vi "Config to String.vi"(8 "error in (no error)":errorcluster, 11 "queue in":T1) -> (0 "error out":errorcluster, 2 "String":string, 3 "queue out":T1)   [LabVIEW 2020, in "NI_LVConfig.lvlib"]
uses:
  NI_LVConfig.lvlib
  Config Queue.ctl
  Config Data.ctl
  Section.ctl
  8.6CompatibleGlobalVar.vi
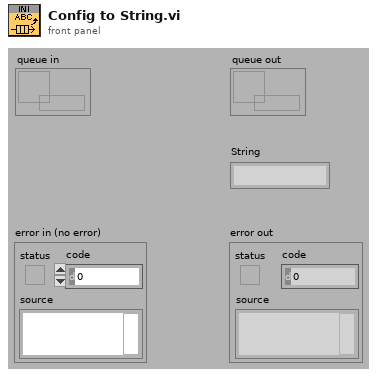
[diagram p1: front panel]
types:
  T1 = typedef "NI_LVConfig.lvlib/Config Queue.ctl" = refnum<queue>
  T2 = typedef "NI_LVConfig.lvlib/Config Data.ctl" = cluster{"sections":T3[], "path":path, "dirty":bool}
  T3 = typedef "NI_LVConfig.lvlib/Section.ctl" = cluster{"name":string, "comment":string, "kvc":string[][]}
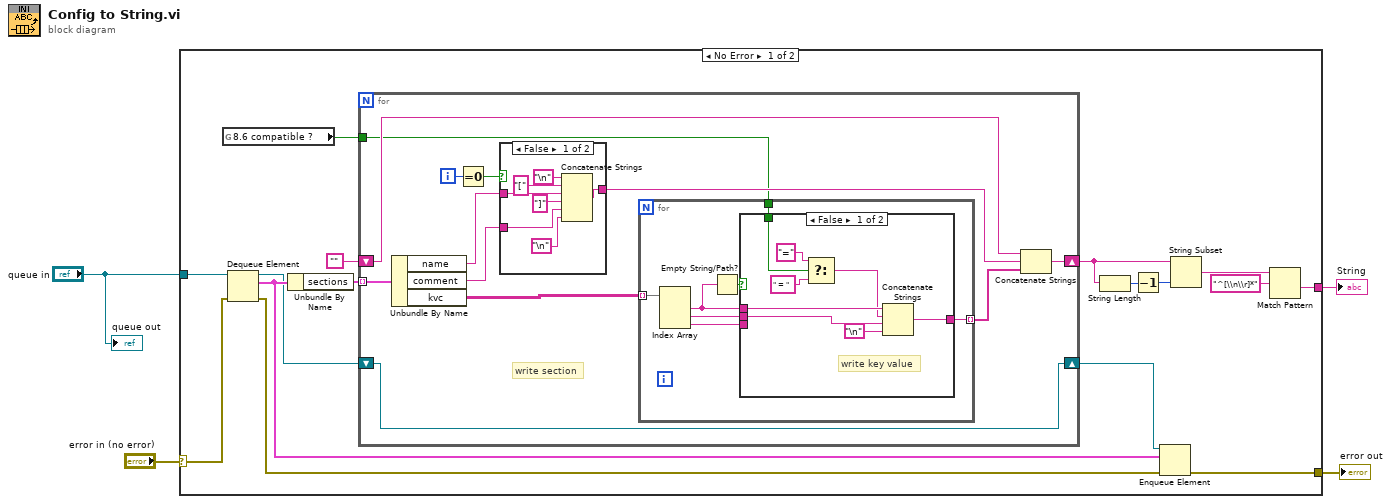
[diagram p0: block diagram]
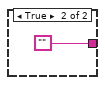
[diagram p2: hidden frame]
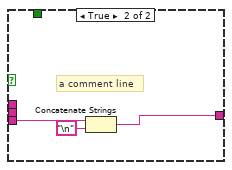
[diagram p3: hidden frame]
diagram:
  n1 = case shown="No Error" "error in (no error)" {
    selector: "error in (no error)" -> [w18 w59]
    tunnel: "queue in" -> [w19 _]
    tunnel: [w15 _] -> w4
    tunnel: [w9 w59] -> w2
    frame No Error {
      n2 = global read "8.6CompatibleGlobalVar.vi" "8.6 compatible ?"() -> (w5:bool)
      n3 = Dequeue Element(queue=w19, error in (no error)=w18) -> (queue out=w7:T1, element=w8:T2, error out=w10:errorcluster)  [unwired: 1 in, 1 out]
      n4 = Unbundle By Name(w8) -> ("sections"=w20:T3[])
      n5 = for {
        tunnel: w20 -> [w32] mode=indexing
        shift-right: [w30] -> w12
        shift-left: "" -> [w29]
        shift-right: [w22] -> w6
        shift-left: w7 -> [w22]
        tunnel: w5 -> [w21]
        i -> [w27]
        # "write section"
        n6 = Unbundle By Name(w32) -> ("name"=w28:string, "comment"=w23:string, "kvc"=w24:string[][])
        n7 = Equal To 0?(x=w27) -> (x = 0?=w26:bool)
        n8 = case shown="False" w26 {
          tunnel: w28 -> [w37 _]
          tunnel: [w36 ""] -> w31
          tunnel: w23 -> [w34 _]
          frame False {
            n9 = Concatenate Strings("\n", "[" ("string"), w37, "]" ("string"), w34, "\n") -> (w36:string)
          }
          frame True {
          }
        }
        n10 = for {
          tunnel: w24 -> [w47] mode=indexing
          tunnel: [w44] -> w25 mode=indexing
          tunnel: w21 -> [w41]
          n11 = Index Array(array=w47) -> (element #1=w42:string, element #2=w43:string, element #3=w45:string)  [unwired: 3 in]
          n12 = Empty String/Path?(string/path=w42) -> (empty?=w46:bool)
          n13 = case shown="False" w46 {
            tunnel: w45 -> [_ w58]
            tunnel: [w52 w56] -> w44
            tunnel: w43 -> [w54 _]
            tunnel: w42 -> [w55 _]
            tunnel: w41 -> [w48 _]
            frame False {
              # "write key value"
              n14 = Select(t="=" ("string"), s=w48, f=" = " ("string")) -> (s? t:f=w49:string)
              n15 = Concatenate Strings(w55, w49, w54, "\n") -> (w52:string)
            }
            frame True {
              # "a comment line"
              n16 = Concatenate Strings(w58, "\n") -> (w56:string)
            }
          }
        }
        n17 = Concatenate Strings(w29, w31, w25) -> (w30:string)
      }
      n18 = String Length(string=w12) -> (length=w14:i32)
      n19 = Decrement(x=w14) -> (x-1=w13:i32)
      n20 = Enqueue Element(queue=w6, element=w8, error in (no error)=w10) -> (error out=w9:errorcluster)  [unwired: 1 in, 2 out]
      n21 = String Subset(string=w12, length (rest)=w13) -> (substring=w11:string)  [unwired: 1 in]
      n22 = Match Pattern(string=w11, regular expression="^[\\n\\r]*") -> (after substring=w15:string)  [unwired: 1 in, 3 out]
    }
    frame Error {
    }
  }
  "error out" <- w2
  "String" <- w4
  "queue out" <- "queue in"
